vi "界面设计.vi"() -> ()   [LabVIEW 2017]
panel:
  in  "主要控制界面":enum32{"实时图像", "校准图样", "追踪数据", "设置"}(tab)
  out "力值估算":dbl[unit]
  out "往返测量":bool
  out "测量中":bool
  out "当前力值计算":dbl[unit]
  out "磁铁终点":dbl[unit]
  out "磁铁起点":dbl[unit]
  out "队列积压数据":u8(slide) scale=0.0..100.0
  out "测量模式":string
  out "文件存放路径":string
  out "测量进度":u8(slide) scale=0.0..100.0
  in  "当前温度":dbl
  in  "磁铁转数":dbl
  in  "磁铁位置":dbl
  in  "焦平面位置":dbl
  out "波形图":dbl[](graph)
  in  "磁球编号":dbl
  out "强度图":dbl[][](graph)
  out "D(Y)":dbl
  out "Y方向均值":dbl
  out "D(X)":dbl
  out "X方向均值":dbl
  out "Z_RMSE":dbl
  out "Z方向均值":dbl
  in  "参考磁球编号":enum16{""}(ring)
  in  "测量磁球编号":enum16{""}(ring)
  out "波形图表":dbl(graph)
  out "采样频率":dbl
  out "数据更新频率":dbl
  in  "旋转电机驱动":bool
  in  "步进电机驱动":bool
  in  "CCD相机驱动":bool
  out "单位像素大小":dbl[unit]
  in  "ROI size":enum16{"64 ", "128"}(ring)
  in  "显微镜放大倍数":dbl
  # "实验信息"
  # "数据监测"
  # "磁铁设置"
  # "驱动设置"
  # "ROI设置"
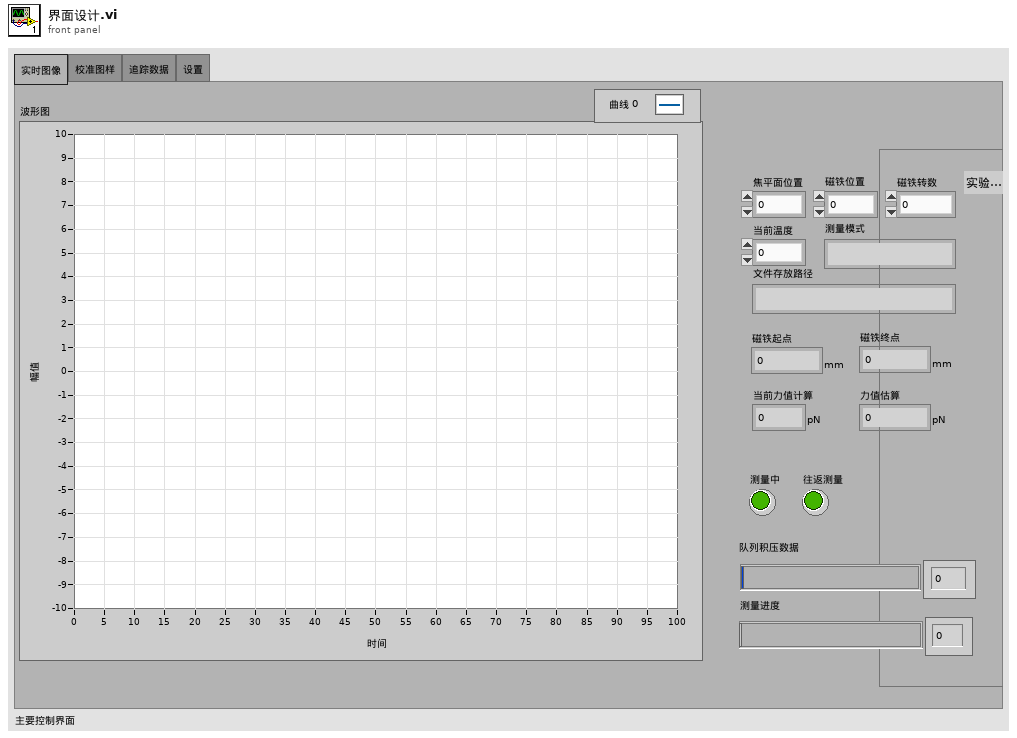
[diagram p1: front panel]
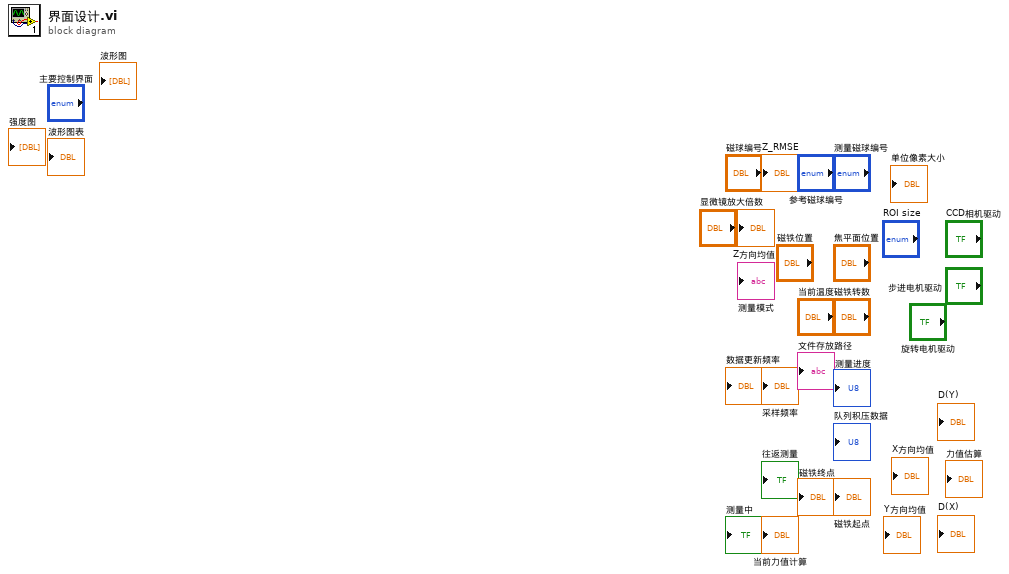
[diagram p0: block diagram]
diagram:
